vi "DB - Array to Columns.vi"(10 "Exclude []":bool, 11 "Array":string[](array[string])) -> (3 "[Columns]":string)   [LabVIEW 2020]
panel:
  # "abc\ndef\nghi"
  # "="
  # "[abc] ,[def] ,[ghi]"
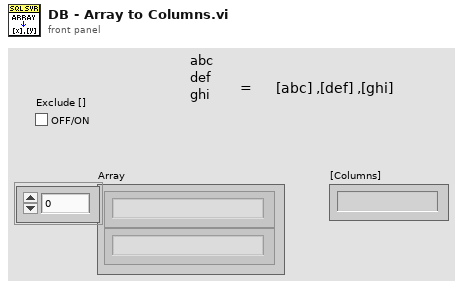
[diagram p1: front panel]
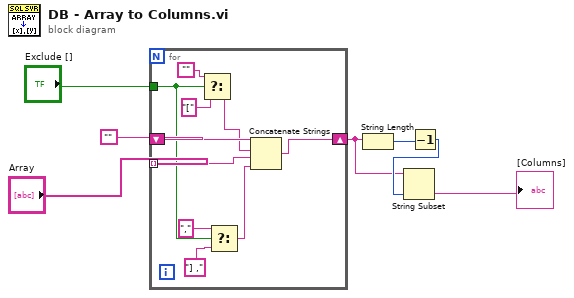
[diagram p0: block diagram]
diagram:
  n1 = for {
    shift-right: [w15] -> w3
    shift-left: "" -> [w17]
    tunnel: "Array" -> [w16] mode=indexing
    tunnel: "Exclude []" -> [w14]
    n2 = Select(t="", s=w14, f="[") -> (s? t:f=w10:string)
    n3 = Select(t=",", s=w14, f="] ,") -> (s? t:f=w12:string)
    n4 = Concatenate Strings(w17, w10, w16, w12) -> (w15:string)
  }
  n5 = String Length(string=w3) -> (length=w4:i32)
  n6 = Decrement(x=w4) -> (x-1=w5:i32)
  n7 = String Subset(string=w3, length (rest)=w5) -> (substring=→"[Columns]":string)  [unwired: 1 in]
